vi "Read DS402 Drive VARs.vi"(7 "R/W Case":T7, 8 "error in (no error)":errorcluster, 9 "Output FIFO buffer in":dbl[](array[numeric]), 10 "I/O Output Data In":T1 {"BD Refs"."Data Reference" format="%.0x"}, 11 "I/O Output Vars in":T4[](array[typedef]) {"VS ref" format="%.0x"}) -> (0 "error out":errorcluster, 1 "Output FIFO buffer out":dbl[](array[numeric]), 2 "I/O Output Data Out":T1 {"BD Refs"."Data Reference" format="%.0x"}, 3 "I/O Output Vars out":T4[](array[typedef]) {"VS ref" format="%.0x"})   [LabVIEW 2016, in "Scan Engine Custom Device.lvlib"]
uses:
  Scan Engine Custom Device.lvlib
  Type Defs/RW Case.ctl
  Type Defs/DS402 Drive ECAT Slave IOV Cluster.ctl
  <vilib>/NI Veristand/Custom Device API/Custom Device Item Ref.ctl
  Type Defs/UDV Data Type.ctl
  Type Defs/Output Data.ctl
  <vilib>/NI Veristand/Custom Device API/Block Data Reference.ctl
  <vilib>/NI Veristand/Custom Device API/Data Reference.ctl
  <vilib>/NI Veristand/Custom Device API/Global Data Refs.vi
  <vilib>/NI Veristand/Custom Device API/Custom Device API.lvlib
  <vilib>/NI Veristand/Custom Device Tools/Custom Device Utility Library/Custom Device Utility Library.lvlib
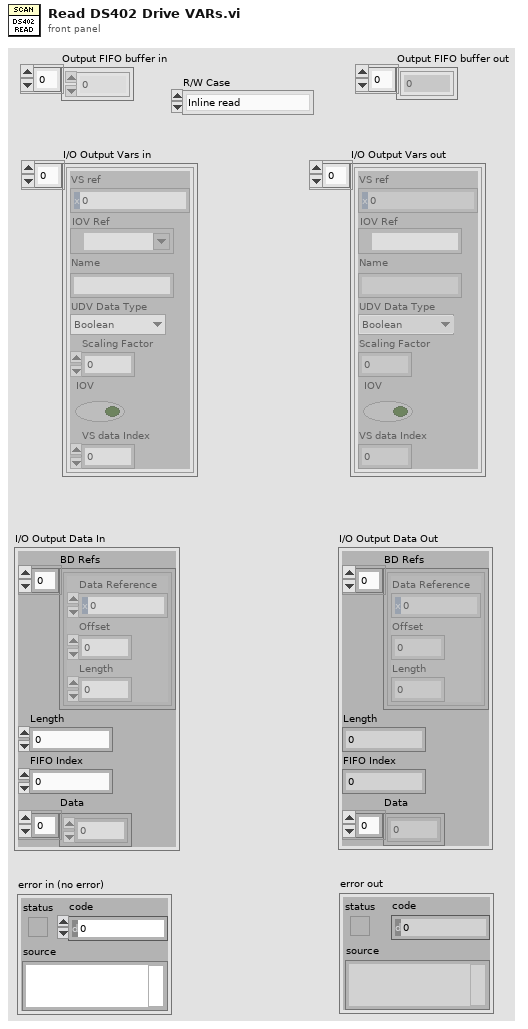
[diagram p1: front panel]
types:
  T1 = typedef "Scan Engine Custom Device.lvlib/Output Data.ctl" = cluster{"BD Refs":T2[], "Length":i32, "FIFO Index":i32, "Data":dbl[]}
  T2 = typedef "Custom Device API.lvlib/Block Data Reference.ctl" = cluster{"Data Reference":T3, "Offset":u64, "Length":u64}
  T3 = typedef "Custom Device API.lvlib/Data Reference.ctl" = i32
  T4 = typedef "Scan Engine Custom Device.lvlib/DS402 Drive ECAT Slave IOV Cluster.ctl" = cluster{"VS ref":T5, "IOV Ref":refnum<k21>, "Name":string, "UDV Data Type":T6, "Scaling Factor":dbl, "IOV":bool, "VS data Index":i32}
  T5 = typedef "Custom Device API.lvlib/Custom Device Item Ref.ctl" = u64
  T6 = typedef "Scan Engine Custom Device.lvlib/UDV Data Type.ctl" = enum16{"Boolean", "Fixed Point", "Int8", "Int16", "Int32", "Int64", "U32 Bit Field", "UInt8", "UInt16", "UInt32", "UInt64", "Other"}
  T7 = typedef "Scan Engine Custom Device.lvlib/RW Case.ctl" = enum16{"Inline read", "Inline write", "Async - Inline loop read", "Async - Inline loop write", "Async loop (read/write)"}
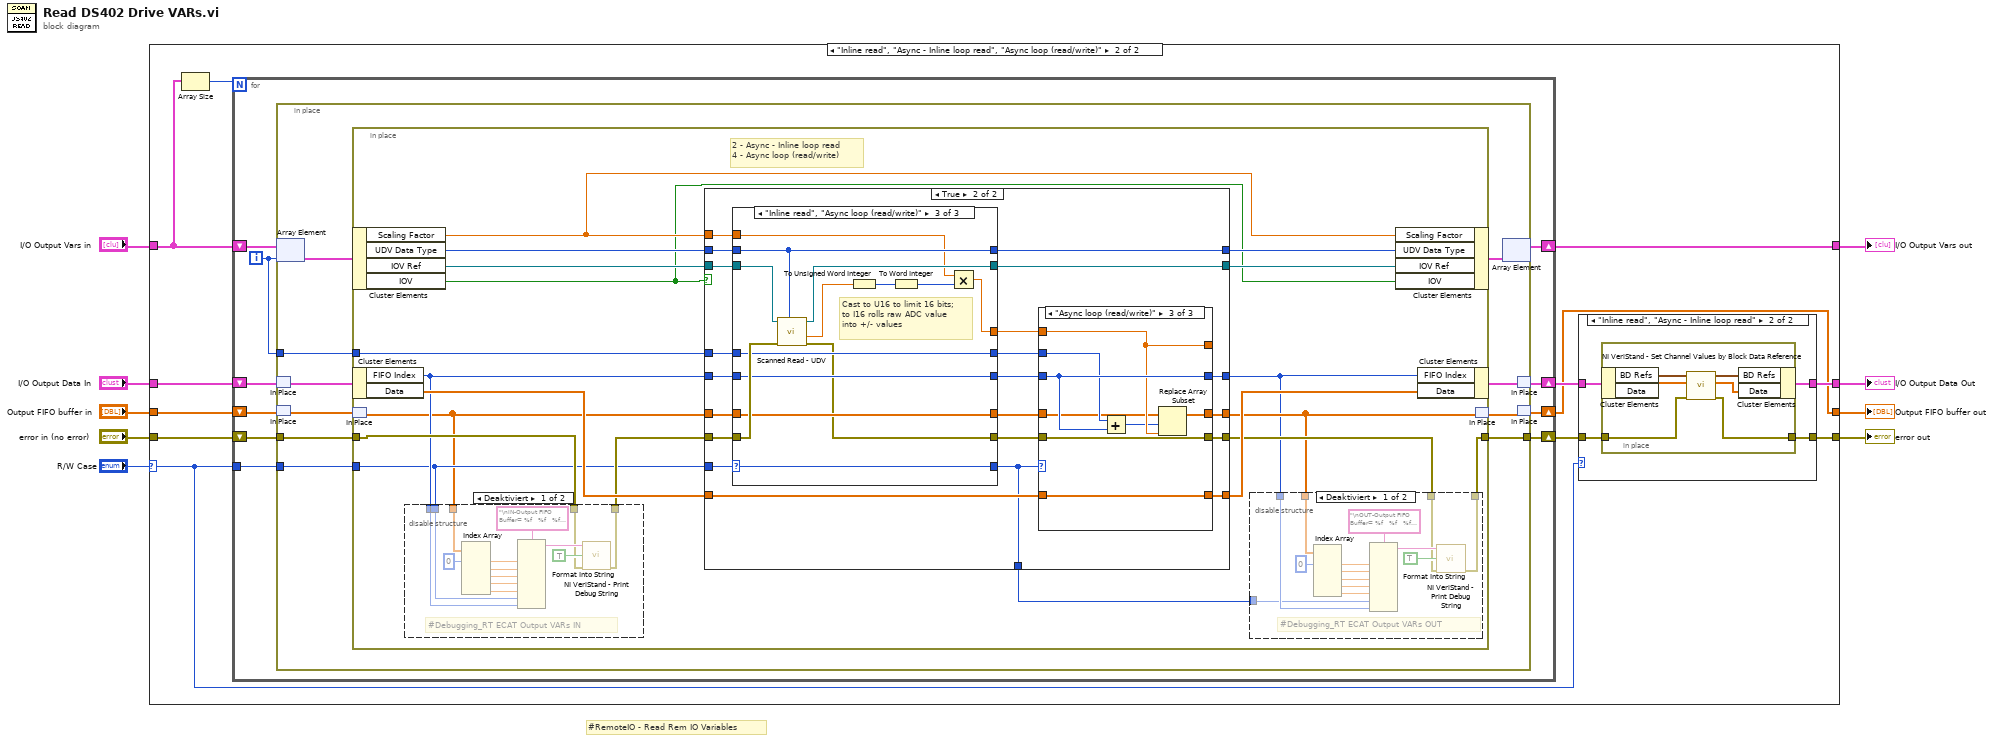
[diagram p0: block diagram]
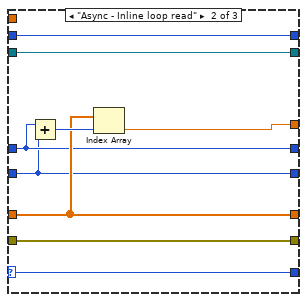
[diagram p5: hidden frame]
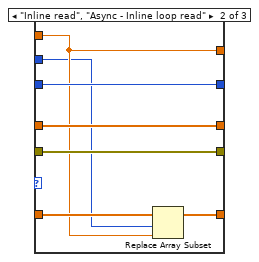
[diagram p7: hidden frame]
diagram:
  # "#RemoteIO - Read Rem IO Variables"
  n1 = case shown="\"Inline read\", \"Async - Inline loop read\", \"Async loop (read/write)\"" "R/W Case" {
    selector: "R/W Case" -> [_ w18]
    tunnel: [w11 w14] -> w9
    tunnel: "Output FIFO buffer in" -> [w11 w25]
    tunnel: [w12 w15] -> w1
    tunnel: [w13 w24] -> w3
    tunnel: "I/O Output Data In" -> [w12 w23]
    tunnel: "I/O Output Vars in" -> [w13 w22]
    tunnel: [w10 w16] -> w7
    tunnel: "error in (no error)" -> [w10 w20]
    frame Default {
    }
    frame "Inline read", "Async - Inline loop read", "Async loop (read/write)" {
      n2 = Array Size(array=w22) -> (size(s)=w21:i32)
      n3 = for {
        N: w21 -> [_]
        shift-right: [w34] -> w24
        shift-left: w22 -> [w35]
        shift-right: [w26] -> w19
        shift-left: w23 -> [w29]
        shift-right: [w32] -> w14
        shift-left: w25 -> [w33]
        shift-right: [w30] -> w17
        shift-left: w20 -> [w31]
        tunnel: w18 -> [w28]
        i -> [w27]
        n4 = in-place {
          in-place-border: w31 -> [w43]
          in-place-border: [w37] -> w30
          in-place-border: w28 -> [w42]
          in-place-border: w27 -> [w41]
          n5 = in-place-array #1(w35, w27) -> (w36:T4)
          n6 = in-place-match #2(w29) -> (w45:T1)
          n7 = in-place-match #3(w33) -> (w44:dbl[])
          n8 = in-place {
            in-place-border: w43 -> [w58]
            in-place-border: w42 -> [w55]
            in-place-border: w41 -> [w61]
            in-place-border: [w52] -> w37
            # "2 - Async - Inline loop read\n4 - Async loop (read/write)"
            n9 = in-place-cluster #4(w36) -> ("Scaling Factor"=w47:dbl, "UDV Data Type"=w63:T6, "IOV Ref"=w62:refnum<k21>, "IOV"=w46:bool)
            n10 = in-place-cluster #5(w45) -> ("FIFO Index"=w56:i32, "Data"=w64:dbl[])
            n11 = in-place-match #6(w44) -> (w54:dbl[])
            n12 = disable-structure shown="Deaktiviert" {
              disable-tunnel: w58 -> [w162 w172]
              disable-tunnel: [w161 w172] -> w57
              disable-tunnel: w56 -> [w160 _]
              disable-tunnel: w55 -> [w159 _]
              disable-tunnel: w54 -> [w158 _]
              frame Disabled {
                # "#Debugging_RT ECAT Output VARs IN"
                n13 = Index Array(array=w158, index #1=0) -> (element #1=w166:dbl, element #2=w165:dbl, element #3=w164:dbl, element #4=w163:dbl, element #5=w171:dbl)  [unwired: 4 in]
                n14 = Format Into String(format string="\nIN-Output FIFO Buffer= %f   %f   %f   %f   %f   - MODE: %d  - Index: %d\n" ("Format-String"), w166, w165, w164, w163, w171, w159, w160) -> (resulting string=w169:string)  [unwired: 2 in, 1 out]
                n15 = call <vilib>:"NI VeriStand - Print Debug String.vi"("error in (no error)"=w162, "Add to log file? (T)"=TRUE, "Message"=w169) -> ("error out"=w161:errorcluster)  [unwired: 8 in]
              }
              frame Enabled {
              }
            }
            n16 = case shown="True" w46 {
              tunnel: w64 -> [w66 w92]
              tunnel: w63 -> [w71 w91]
              tunnel: w62 -> [w70 w90]
              tunnel: w61 -> [_ w89]
              tunnel: [w71 w88] -> w60
              tunnel: [w66 w84] -> w59
              tunnel: w57 -> [w67 w83]
              tunnel: w56 -> [w69 w82]
              tunnel: w55 -> [w65 w81]
              tunnel: w54 -> [w68 w80]
              tunnel: [w67 w79] -> w53
              tunnel: [w68 w78] -> w51
              tunnel: [w69 w77] -> w50
              tunnel: [w65 w76] -> w49
              tunnel: [w70 w73] -> w48
              tunnel: w47 -> [_ w72]
              frame False {
              }
              frame True {
                n17 = case shown="\"Inline read\", \"Async loop (read/write)\"" w81 {
                  selector: w81 -> [w93 w103 w114]
                  tunnel: w91 -> [w94 w101 w115]
                  tunnel: w90 -> [w95 w102 w122]
                  tunnel: w82 -> [w97 w104 w118]
                  tunnel: w80 -> [w98 w107 w117]
                  tunnel: [w98 w107 w117] -> w85
                  tunnel: w89 -> [w96 w105 w119]
                  tunnel: [_ w106 w113] -> w75
                  tunnel: [w96 w105 w119] -> w87
                  tunnel: [w97 w104 w118] -> w86
                  tunnel: [w93 w103 w114] -> w76
                  tunnel: [w95 w102 w121] -> w73
                  tunnel: [w94 w101 w115] -> w88
                  tunnel: w83 -> [w99 w100 w120]
                  tunnel: [w99 w100 w116] -> w74
                  tunnel: w72 -> [_ _ w109]
                  frame Default {
                  }
                  frame "Async - Inline loop read" {
                    n18 = Add(x=w105, y=w104) -> (x+y=w108:i32)
                    n19 = Index Array(array=w107, index=w108) -> (element=w106:dbl)
                  }
                  frame "Inline read", "Async loop (read/write)" {
                    # "Cast to U16 to limit 16 bits;\nto I16 rolls raw ADC value\ninto +/- values"
                    n20 = call "Scanned Read - UDV.vi"("UDV Data Type"=w115, "error in (no error)"=w120, "IOV ref in"=w122) -> ("error out"=w116:errorcluster, "data out"=w112:dbl, "IOV ref out"=w121:refnum<k21>)  [unwired: 6 in]
                    n21 = To Unsigned Word Integer(number=w112) -> (unsigned 16bit integer=w110:u16)
                    n22 = To Word Integer(number=w110) -> (16bit integer=w111:i16)
                    n23 = Multiply(x=w109, y=w111) -> (x*y=w113:dbl)
                  }
                }
                n24 = case shown="\"Async loop (read/write)\"" w76 {
                  tunnel: w87 -> [_ w128 w138]
                  tunnel: w86 -> [w123 w130 w139]
                  tunnel: w75 -> [w124 w129 w137]
                  tunnel: w85 -> [w125 w131 w136]
                  tunnel: w74 -> [w126 w132 w141]
                  tunnel: w92 -> [w127 w134 w140]
                  tunnel: [w123 w130 w139] -> w77
                  tunnel: [w127 w133 w140] -> w84
                  tunnel: [w126 w132 w141] -> w79
                  tunnel: [w125 w131 w142] -> w78
                  tunnel: [w124 w129 w137] -> _
                  frame Default {
                  }
                  frame "Inline read", "Async - Inline loop read" {
                    n25 = Replace Array Subset(array=w134, new element=w129, index=w128) -> (w133:dbl[])
                  }
                  frame "Async loop (read/write)" {
                    n26 = Add(x=w138, y=w139) -> (x+y=w135:i32)
                    n27 = Replace Array Subset(array=w136, new element=w137, index=w135) -> (w142:dbl[])
                  }
                }
              }
            }
            n28 = disable-structure shown="Deaktiviert" {
              disable-tunnel: w53 -> [w147 w157]
              disable-tunnel: [w146 w157] -> w52
              disable-tunnel: w51 -> [w145 _]
              disable-tunnel: w50 -> [w144 _]
              disable-tunnel: w49 -> [w143 _]
              frame Disabled {
                # "#Debugging_RT ECAT Output VARs OUT"
                n29 = Index Array(array=w145, index #1=0) -> (element #1=w151:dbl, element #2=w150:dbl, element #3=w149:dbl, element #4=w148:dbl, element #5=w156:dbl)  [unwired: 4 in]
                n30 = Format Into String(format string="\nOUT-Output FIFO Buffer= %f   %f   %f   %f   %f   - MODE: %d  - Index: %d\n" ("Format-String"), w151, w150, w149, w148, w156, w143, w144) -> (resulting string=w154:string)  [unwired: 2 in, 1 out]
                n31 = call <vilib>:"NI VeriStand - Print Debug String.vi"("error in (no error)"=w147, "Add to log file? (T)"=TRUE, "Message"=w154) -> ("error out"=w146:errorcluster)  [unwired: 8 in]
              }
              frame Enabled {
              }
            }
            n32 = in-place-cluster #4("Scaling Factor"=w47, "UDV Data Type"=w60, "IOV Ref"=w48, "IOV"=w46) -> (w40:T4)
            n33 = in-place-cluster #5("FIFO Index"=w50, "Data"=w59) -> (w39:T1)
            n34 = in-place-match #6(w51) -> (w38:dbl[])
          }
          n35 = in-place-array #1(w40) -> (w34:T4[])  [unwired: 1 out]
          n36 = in-place-match #2(w39) -> (w26:T1)
          n37 = in-place-match #3(w38) -> (w32:dbl[])
        }
      }
      n38 = case shown="\"Inline read\", \"Async - Inline loop read\"" w18 {
        tunnel: w19 -> [w173 w175]
        tunnel: w17 -> [w174 w178]
        tunnel: [w174 w177] -> w16
        tunnel: [w173 w176] -> w15
        frame Default {
        }
        frame "Inline read", "Async - Inline loop read" {
          n39 = in-place {
            in-place-border: w178 -> [w182]
            in-place-border: [w181] -> w177
            n40 = in-place-cluster #7(w175) -> ("BD Refs"=w180:T2[], "Data"=w179:dbl[])
            n41 = call <vilib>:"NI VeriStand - Set Channel Values by Block Data Reference.vi"("error in (no error)"=w182, "Values Array in"=w179, "Block Data Ref"=w180) -> ("error out"=w181:errorcluster, "Values Array out"=w183:dbl[], "Block Data Ref dup"=w184:T2[])  [unwired: 6 in]
            n42 = in-place-cluster #7("BD Refs"=w184, "Data"=w183) -> (w176:T1)
          }
        }
      }
    }
  }
  "Output FIFO buffer out" <- w9
  "error out" <- w7
  "I/O Output Vars out" <- w3
  "I/O Output Data Out" <- w1
